vi "XML_FAIL_Iteme.vi"(0 "组合框":string(combo)="Double", 1 "Name":string, 2 "UpperLimit":string, 3 "Value":string, 4 "LowerLimit":string, 5 "MeasurementUnit":string, 6 "StatusCode":string) -> (20 "连接的字符串":string)   [LabVIEW 2018]
uses:
  Subvi/Global.vi
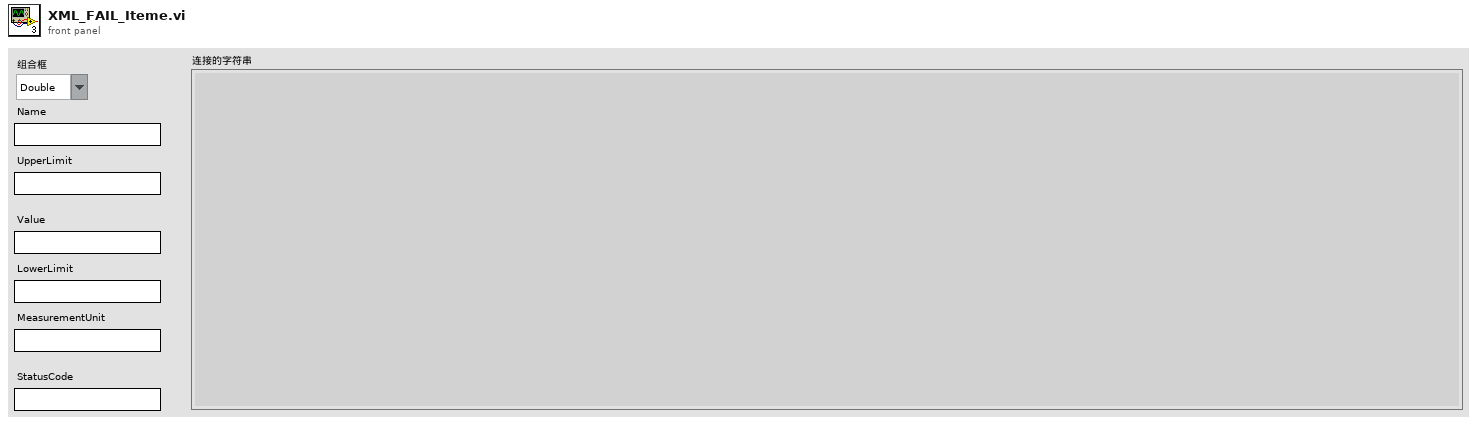
[diagram p1: front panel]
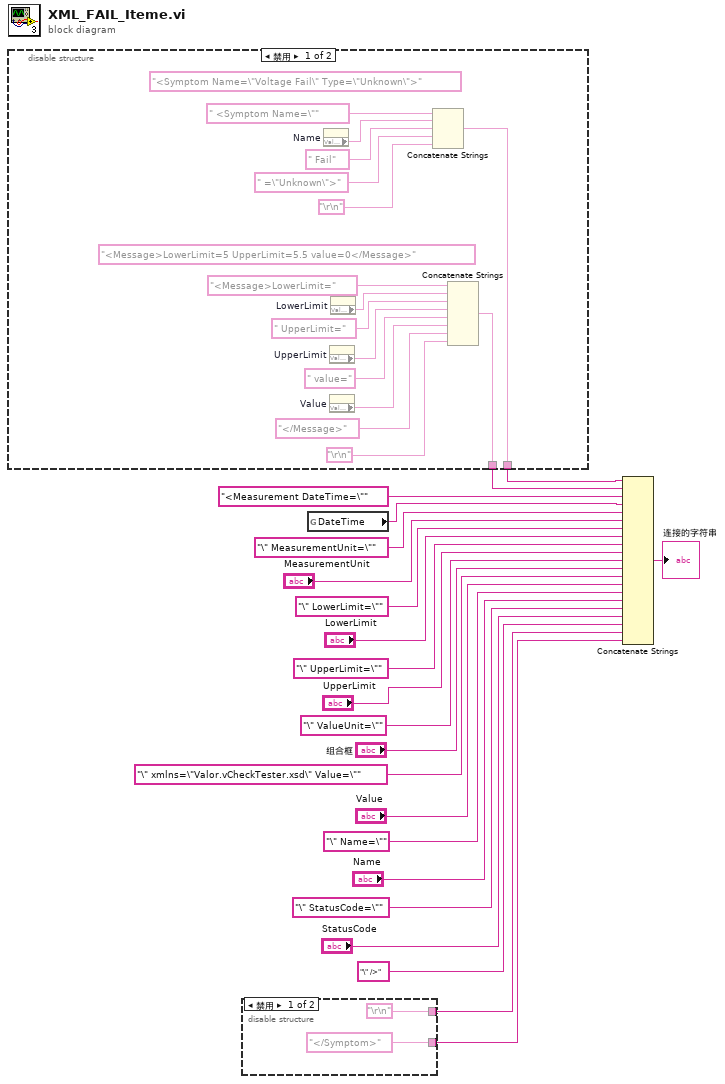
[diagram p0: block diagram]
diagram:
  n1 = disable-structure shown="禁用" {
    disable-tunnel: [w26 _] -> w3
    disable-tunnel: [w25 _] -> w2
    frame Disabled {
      (unwired) "<Message>LowerLimit=5 UpperLimit=5.5 value=0</Message>"
      (unwired) "<Symptom Name=\"Voltage Fail\" Type=\"Unknown\">"
      n2 = property on="Name" class="Str"() -> ("Value"=w36:string)  [unwired: 2 in, 2 out]
      n3 = property on="UpperLimit" class="Str"() -> ("Value"=w30:string)  [unwired: 2 in, 2 out]
      n4 = property on="Value" class="Str"() -> ("Value"=w28:string)  [unwired: 2 in, 2 out]
      n5 = property on="LowerLimit" class="Str"() -> ("Value"=w32:string)  [unwired: 2 in, 2 out]
      n6 = Concatenate Strings(" <Symptom Name=\"", w36, " Fail", " =\"Unknown\">", "\r\n") -> (w25:string)
      n7 = Concatenate Strings("<Message>LowerLimit=", w32, " UpperLimit=", w30, " value=", w28, "</Message>", "\r\n") -> (w26:string)
    }
    frame Enabled {
    }
  }
  n8 = disable-structure shown="禁用" {
    disable-tunnel: ["\r\n" _] -> w4
    disable-tunnel: ["</Symptom>" _] -> w1
    frame Disabled {
    }
    frame Enabled {
    }
  }
  n9 = global read "Global.vi" "DateTime"() -> (w21:string)
  n10 = Concatenate Strings(w2, w3, "<Measurement DateTime=\"", w21, "\" MeasurementUnit=\"", "MeasurementUnit", "\" LowerLimit=\"", "LowerLimit", "\" UpperLimit=\"", "UpperLimit", "\" ValueUnit=\"", "组合框", "\" xmlns=\"Valor.vCheckTester.xsd\" Value=\"", "Value", "\" Name=\"", "Name", "\" StatusCode=\"", "StatusCode", "\" />", w4, w1) -> (→"连接的字符串":string)
